vi "Set Available Entities.vi"(10 "Available Entities":T1[](array[typedef]), 11 "RelationPanel in":refnum<class "RelationPanel.lvclass">) -> (3 "RelationPanel out":refnum<class "RelationPanel.lvclass">)   [LabVIEW 2020, in "Conditum-Tools.lvlib" / "RelationPanel.lvclass"]
uses:
  RelationPanel.lvclass
  Available Entity.ctl
  RelationPanel.lvclass/RelationPanel.ctl
  Conditum-Tools.lvlib
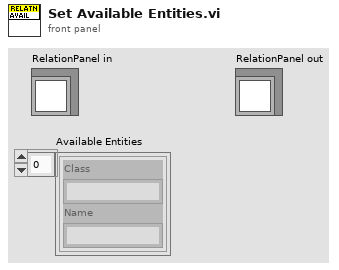
[diagram p1: front panel]
types:
  T1 = typedef "Conditum-Tools.lvlib/Available Entity.ctl" = cluster{"Class":string, "Name":string}
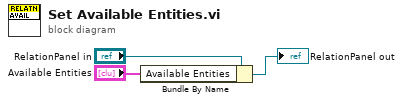
[diagram p0: block diagram]
diagram:
  n1 = Bundle By Name(cluster="RelationPanel in", "Available Entities"="Available Entities") -> (→"RelationPanel out":refnum<class "RelationPanel.lvclass">)
